vi "Write String.vi"(8 "error in (no error)":errorcluster, 10 "Abs_String.lvclass":refnum<class "Abs_String.lvclass">, 11 "StringLen_I32 in":refnum<class "StringLen_I32.lvclass">) -> (0 "error out":errorcluster, 3 "StringLen_I32 out":refnum<class "StringLen_I32.lvclass">)   [LabVIEW 2021, in "StringLen_I32.lvclass"]
uses:
  StringLen_I32.lvclass
  Abs_Types/String/Abs_String.lvclass
  StringLen_I32.lvclass/StringLen_I32.ctl
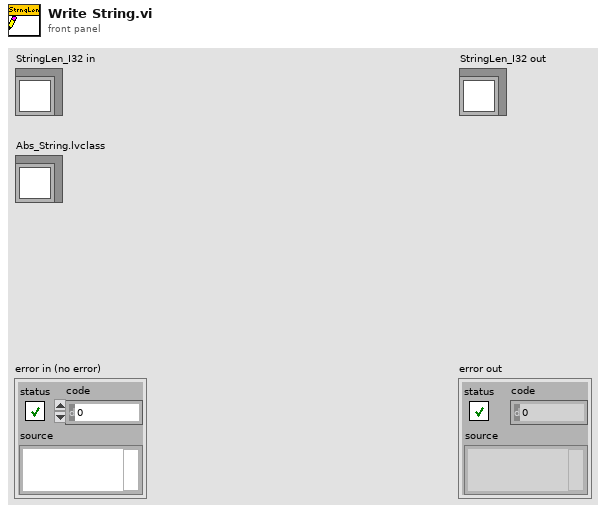
[diagram p1: front panel]
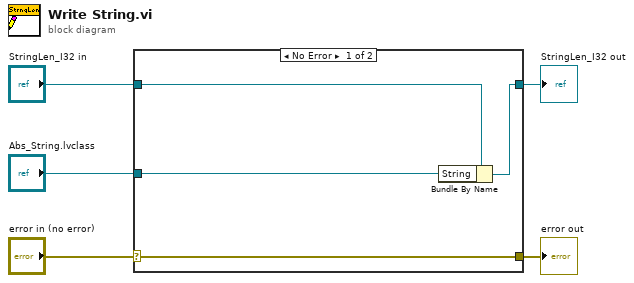
[diagram p0: block diagram]
diagram:
  n1 = case shown="No Error" "error in (no error)" {
    selector: "error in (no error)" -> [w9 w10]
    tunnel: [w9 w10] -> w4
    tunnel: [w7 w11] -> w2
    tunnel: "StringLen_I32 in" -> [w8 w11]
    tunnel: "Abs_String.lvclass" -> [w6 _]
    frame No Error {
      n2 = Bundle By Name(cluster=w8, "String"=w6) -> (w7:refnum<class "StringLen_I32.lvclass">)
    }
    frame Error {
    }
  }
  "error out" <- w4
  "StringLen_I32 out" <- w2
